vi "Read Trace.vi"(8 "error in (no error)":errorcluster, 9 "Maximum Time (10000)":u32=10000, 11 "VISA resource name":refnum<visa-resource-name>) -> (0 "error out":errorcluster, 2 "Trace Waveform":T1(graph), 3 "VISA resource name out":refnum<visa-resource-name>)   [LabVIEW 2020, in "Template - Spectrum Analyzer.lvlib"]
doc: "Reads a trace from the spectrum analyzer."
uses:
  <instrlib>/_Template - Spectrum Analyzer/Template - Spectrum Analyzer.lvlib
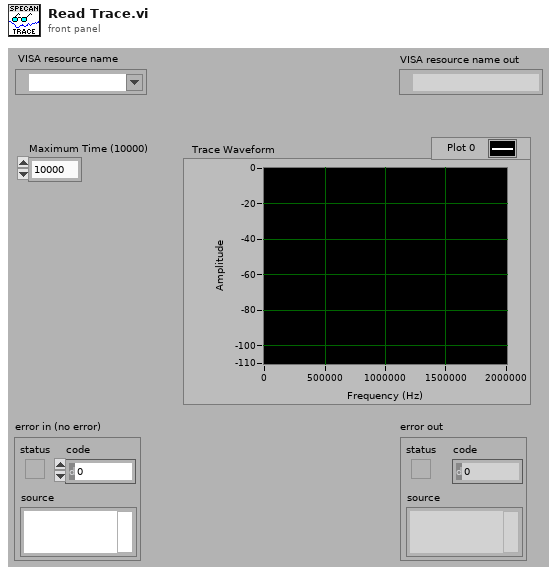
[diagram p1: front panel]
types:
  T1 = cluster{"Start Frequency (0 Hz)":dbl, dbl, "Trace":sgl[]}
  T2 = cluster{"Initial X":dbl, "X Increment":dbl, "Trace Array":sgl[]}
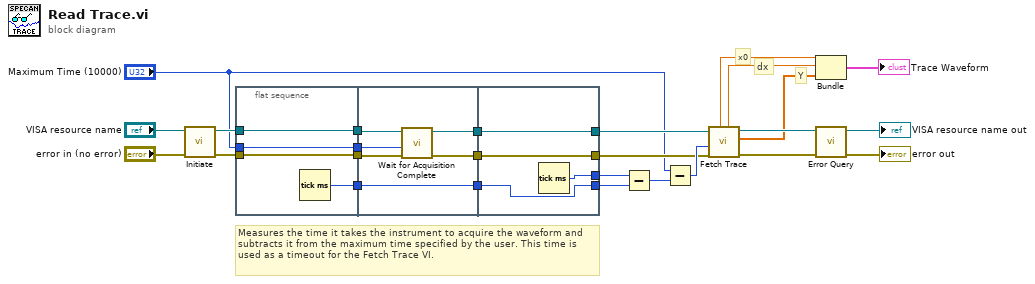
[diagram p0: block diagram]
diagram:
  # "Measures the time it takes the instrument to acquire the waveform and subtracts it from the maximum time specified by the user. This time is used as a timeout for the Fetch Trace VI."
  # "Y"
  # "dx"
  # "x0"
  n1 = call <instrlib>:"Initiate.vi"("error in (no error)"="error in (no error)", "VISA resource name"="VISA resource name") -> ("error out"=w10:errorcluster, "VISA resource name out"=w12:refnum<visa-resource-name>)  [unwired: 8 in]
  n2 = flat-sequence {
    tunnel: [w30] -> w7
    tunnel: w12 -> [w29]
    tunnel: [w29] -> w6
    tunnel: w10 -> [w28]
    tunnel: [w28] -> w5
    tunnel: "Maximum Time (10000)" -> [w27]
    tunnel: [w27] -> w4
    tunnel: w7 -> [w31]
    tunnel: [w31] -> w3
    tunnel: w6 -> [w36]
    tunnel: [w35] -> w2
    tunnel: w5 -> [w34]
    tunnel: [w33] -> w1
    tunnel: w4 -> [w32]
    tunnel: [w39] -> w15
    tunnel: w3 -> [w39]
    tunnel: [w40] -> w14
    tunnel: [w38] -> w11
    tunnel: w2 -> [w38]
    tunnel: [w37] -> w9
    tunnel: w1 -> [w37]
    frame #0 {
      n3 = Tick Count (ms)() -> (millisecond timer value=w30:u32)
    }
    frame #1 {
      n4 = call <instrlib>:"Wait for Acquisition Complete.vi"("error in (no error)"=w34, "Maximum Time (10000)"=w32, "VISA resource name"=w36) -> ("error out"=w33:errorcluster, "VISA resource name out"=w35:refnum<visa-resource-name>)  [unwired: 7 in]
    }
    frame #2 {
      n5 = Tick Count (ms)() -> (millisecond timer value=w40:u32)
    }
  }
  n6 = Subtract(x=w14, y=w15) -> (x-y=w16:u32)
  n7 = Subtract(x="Maximum Time (10000)", y=w16) -> (x-y=w13:u32)
  n8 = call <instrlib>:"Fetch Trace.vi"("error in (no error)"=w9, "Timeout (10000 ms)"=w13, "VISA resource name"=w11) -> ("error out"=w22:errorcluster, "Trace Array"=w17:sgl[], "VISA resource name out"=w24:refnum<visa-resource-name>, "X Increment"=w20:dbl, "Initial X"=w19:dbl)  [unwired: 4 in]
  n9 = Bundle("Initial X"=w19, "X Increment"=w20, "Trace Array"=w17) -> (→"Trace Waveform":T2)  [unwired: 1 in]
  n10 = call <instrlib>:"Error Query.vi"("error in (no error)"=w22, "VISA resource name"=w24) -> ("error out"=→"error out":errorcluster, "VISA resource name out"=→"VISA resource name out":refnum<visa-resource-name>)  [unwired: 6 in, 2 out]
